vi "Out_Off_F5xxx.vi"(4 "Driver Name":T8, 5 "SwitchOFF":bool=TRUE, 6 "Error Code":T9, 7 "Model":T6, 8 "error in":T7, 11 "DriverConnect in":T1={"InterfaceType"=enum."VISA", "OpenedSession"="", "InterfaceSettings"={"Interface"=enum."RS232", "EOS 4 read"=enum."LF (\\n)", "EOS 4 write"=enum."LF (\\n)", "TMO, ms"=10000, "Sett"=variant(cluster{"Baud Rate":u32, "Data Bits":u16, "Parity":u16, "Stop Bits":u16, "Flow Control":u16, "Eho":bool} {"Baud Rate"=75, "Data Bits"=0, "Parity"=0, "Stop Bits"=0, "Flow Control"=0, "Eho"=FALSE})}}) -> (0 "error out":T7, 3 "DriverConnect out":T1={"InterfaceType"=enum."VISA", "OpenedSession"="", "InterfaceSettings"={"Interface"=enum."RS232", "EOS 4 read"=enum."LF (\\n)", "EOS 4 write"=enum."LF (\\n)", "TMO, ms"=10000, "Sett"=variant(cluster{"Baud Rate":u32, "Data Bits":u16, "Parity":u16, "Stop Bits":u16, "Flow Control":u16, "Eho":bool} {"Baud Rate"=75, "Data Bits"=0, "Parity"=0, "Stop Bits"=0, "Flow Control"=0, "Eho"=FALSE})}})   [LabVIEW 2018]
uses:
  MOKO_LabViewLibrary/MokoLowLevel/MokoLowLovelControl/MLLC_ErrorCode.ctl
  MOKO_LabViewLibrary/MokoLowLevel/MokoLowLovelControl/MLLC_DriverName.ctl
  MOKO_LabViewLibrary/MokoLowLevel/MokoLowLovelControl/MLLC_Error.ctl
  Models.ctl
  MOKO_LabViewLibrary/MokoLowLevel/MokoLowLovelControl/MLLC_ConnectCluster.ctl
  MOKO_LabViewLibrary/MokoLowLevel/MokoLowLovelControl/MLLC_InterfaceType.ctl
  MOKO_LabViewLibrary/MokoLowLevel/MokoLowLovelControl/MLLC_OpenedSession.ctl
  MOKO_LabViewLibrary/MokoLowLevel/MokoLowLovelControl/MLLC_InterfaceSettings.ctl
  MOKO_LabViewLibrary/MokoLowLevel/MokoLowLovelControl/MLLC_InterfaceKind.ctl
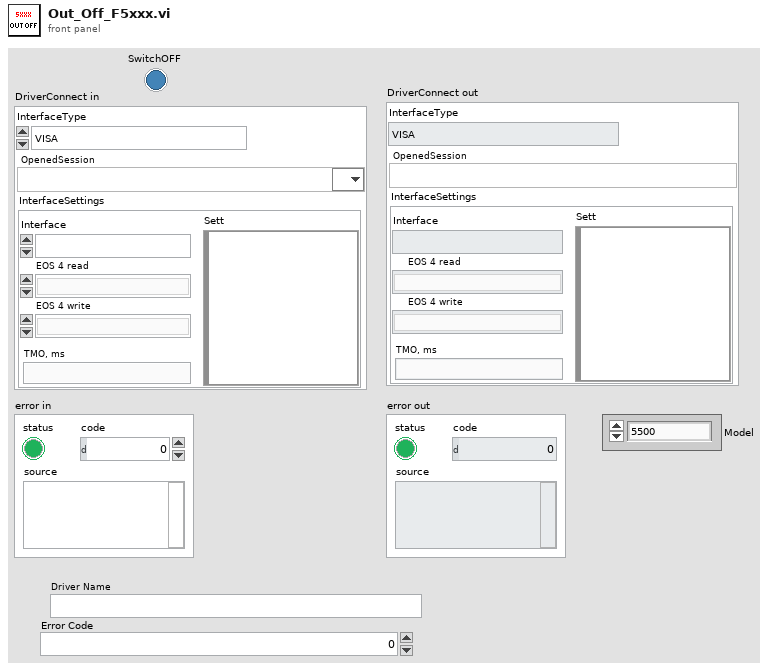
[diagram p1: front panel]
types:
  T1 = typedef "MLLC_ConnectCluster.ctl" = cluster{"InterfaceType":T2, "OpenedSession":T3, "InterfaceSettings":T4}
  T2 = typedef "MLLC_InterfaceType.ctl" = enum16{"VISA", "Prologix USB-GPIB"}
  T3 = typedef "MLLC_OpenedSession.ctl" = refnum<visa-resource-name>
  T4 = typedef "MLLC_InterfaceSettings.ctl" = cluster{"Interface":T5, "EOS 4 read":enum16{"Default (=EOS 4 write)", "CR (\\r)", "LF (\\n)", "None"}, "EOS 4 write":enum16{"CR+LF (\\r\\n)", "CR (\\r)", "LF (\\n)", "None"}, "TMO, ms":i32, "Sett":variant}
  T5 = typedef "MLLC_InterfaceKind.ctl" = enum16{"RS232", "GPIB", "USB", "Ethernet", "another"}
  T6 = typedef "Models.ctl" = enum16{"5500", "5520", "5700", "5720", "5502", "5522", "5730"}
  T7 = typedef "MLLC_Error.ctl" = errorcluster
  T8 = typedef "MLLC_DriverName.ctl" = string
  T9 = typedef "MLLC_ErrorCode.ctl" = u32
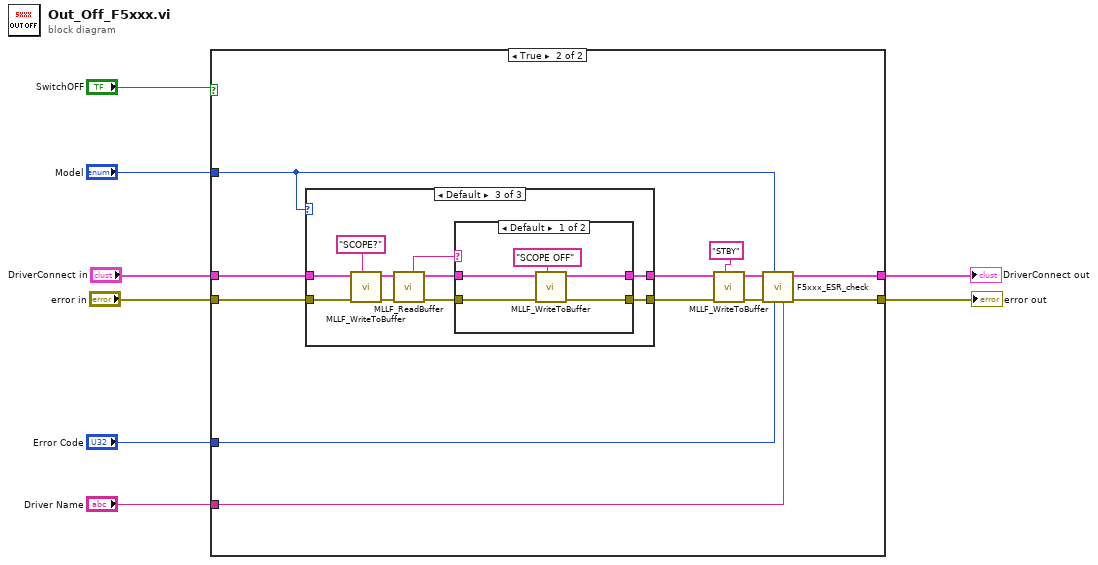
[diagram p0: block diagram]
diagram:
  n1 = case shown="True" "SwitchOFF" {
    tunnel: [w9 w19] -> w1
    tunnel: [w10 w18] -> w8
    tunnel: "Driver Name" -> [_ w17]
    tunnel: "Error Code" -> [_ w16]
    tunnel: "error in" -> [w10 w15]
    tunnel: "Model" -> [_ w13]
    tunnel: "DriverConnect in" -> [w9 w12]
    frame False {
    }
    frame True {
      n2 = case shown="Default" w13 {
        tunnel: w15 -> [w24 w26 w36]
        tunnel: [w24 w26 w29] -> w14
        tunnel: w12 -> [w23 w25 w28]
        tunnel: [w23 w25 w27] -> w11
        frame "5720", "5730" {
        }
        frame "5502" {
        }
        frame Default {
          n3 = call "MLLF_WriteToBuffer.vi"("String"="SCOPE?", "error in"=w36, "DriverConnect in"=w28) -> ("error out"=w34:T7, "DriverConnect out"=w33:T1)  [unwired: 5 in]
          n4 = call "MLLF_ReadBuffer.vi"("Error In"=w34, "DriverConnect in"=w33) -> ("Error Out"=w31:errorcluster, "DriverConnect out"=w32:T1, "String"=w30:string)  [unwired: 6 in]
          n5 = case shown="Default" w30 {
            tunnel: w32 -> [w39 w43]
            tunnel: w31 -> [w40 w42]
            tunnel: [w38 w43] -> w27
            tunnel: [w37 w42] -> w29
            frame Default {
              n6 = call "MLLF_WriteToBuffer.vi"("String"="SCOPE OFF", "error in"=w40, "DriverConnect in"=w39) -> ("error out"=w37:T7, "DriverConnect out"=w38:T1)  [unwired: 5 in]
            }
            frame "OFF" {
            }
          }
        }
      }
      n7 = call "MLLF_WriteToBuffer.vi"("String"="STBY", "error in"=w14, "DriverConnect in"=w11) -> ("error out"=w21:T7, "DriverConnect out"=w20:T1)  [unwired: 5 in]
      n8 = call "F5xxx_ESR_check.vi"("Driver Name"=w17, "Error Code"=w16, "Model"=w13, "error in"=w21, "DriverConnect in"=w20) -> ("error out"=w18:T7, "DriverConnect out"=w19:T1)  [unwired: 5 in]
    }
  }
  "error out" <- w8
  "DriverConnect out" <- w1
